vi "~test dialogs, data structure and Start-build seq VIs.vi"   [LabVIEW 2017]
uses:
  Classes/Sequence/Sequence.lvclass
types:
  T1 = typedef "Mode1TestProperties.ctl" = cluster{"Probe Horizontal Polarization":bool, "Probe Vertical Polarization":bool, "Data File Name":string, "RF In/Out of antenna":T2, "Raster XY Points":cluster{"X mm":dbl, "Y mm":dbl}[]}
  T2 = typedef "RF Direction.ctl" = enum16{"Tx - RF In", "Rx - RF Out"}
  T3 = typedef "mWaveTestStep.ctl" = cluster{"StepType":T4, "RF In/Out":T2, "Module/Raster":i32, "Polarization":T5, "AO-64 Array":dbl[], "Position":cluster{"X mm":dbl, "Y mm":dbl, "Z mm":dbl, "T deg":dbl}}
  T4 = typedef "TestStepTypes.ctl" = enum16{"Patch", "Motion", "SweepTest", "RasterTest", "Finish", "64ModuleCfg"}
  T5 = typedef "PolarizationSelect.ctl" = enum16{"Vertical", "Horizontal"}
  T6 = typedef "Mode2TestProperties.ctl" = cluster{"Probe Horizontal Polarization":bool, "Probe Vertical Polarization":bool, "Upload TR Module file":path, "Data File Name":string, "RF In/Out of antenna":T2, "RT3 Positions, degrees":dbl[]}
  T7 = typedef "Mode3TestProperties.ctl" = cluster{"Probe Horizontal Polarization":bool, "Probe Vertical Polarization":bool, "Upload TR Module file":path, "Data File Name":string, "RF In/Out of antenna":T2}
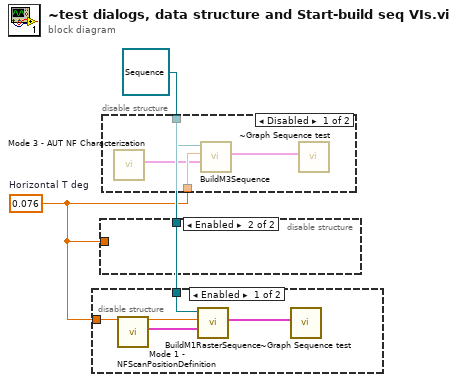
[diagram p0: block diagram]
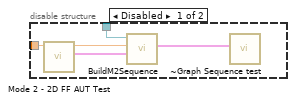
[diagram p2: hidden frame]
diagram:
  w1 = 0.076  # Horizontal T deg
  w2 = refnum<class "Sequence.lvclass"> refnum ("Sequence in")
  n1 = disable-structure shown="Enabled" {
    disable-tunnel: w2 -> [w6 _]
    disable-tunnel: w1 -> [w3 _]
    frame Enabled {
      n2 = call "Mode 1 - NFScanPositionDefinition.vi"() -> ("Mode3TestProperties"=w5:T1)  [unwired: 10 in, 1 out]
      n3 = call "BuildM1RasterSequence.vi"("Mode3TestProperties"=w5, "Horizontal T deg"=w3, "Sequence in"=w6) -> ("PAARD Test Sequence"=w4:T3[])  [unwired: 6 in, 2 out]
      n4 = call "~Graph Sequence test.vi"("PAARD Test Seq"=w4) -> ()  [unwired: 11 in]
    }
    frame Disabled {
    }
  }
  n5 = disable-structure shown="Enabled" {
    disable-tunnel: w2 -> [w10 _]
    disable-tunnel: w1 -> [w9 _]
    frame Disabled {
      n6 = call "Mode 2 - 2D FF AUT Test.vi"() -> ("Mode2 Test Properties"=w8:T6)  [unwired: 10 in, 1 out]
      n7 = call "BuildM2Sequence.vi"("Mode2 Test Properties"=w8, "Horizontal T deg"=w9, "Sequence in"=w10) -> ("PAARD Test Seq"=w7:T3[])  [unwired: 6 in, 2 out]
      n8 = call "~Graph Sequence test.vi"("PAARD Test Seq"=w7) -> ()  [unwired: 11 in]
    }
    frame Enabled {
    }
  }
  n9 = disable-structure shown="Disabled" {
    disable-tunnel: w2 -> [w14 _]
    disable-tunnel: w1 -> [w13 _]
    frame Disabled {
      n10 = call "Mode 3 - AUT NF Characterization.vi"() -> ("Mode3 Test Properties"=w12:T7)  [unwired: 10 in, 1 out]
      n11 = call "BuildM3Sequence.vi"("Mode3 Test Properties"=w12, "Horizontal T deg"=w13, "Sequence in"=w14) -> ("PAARD Test Sequence"=w11:T3[])  [unwired: 6 in, 2 out]
      n12 = call "~Graph Sequence test.vi"("PAARD Test Seq"=w11) -> ()  [unwired: 11 in]
    }
    frame Enabled {
    }
  }
